vi "VI Reference Based Quadrature.vi"() -> ()   [LabVIEW 2023]
doc: "This example VI shows how to use the Quadrature VI to calculate integrals, and compares the integration results and execution time of 1D Quadrature (VI).vi with the integration results and execution time of 1D Quadrature (Formula).vi."
uses:
  <vilib>/Analysis/1siggen.llb/Ramp Pattern by Samples.vi
  <vilib>/Analysis/8numeric.llb/1D Quadrature (VI).vi
  <vilib>/Analysis/8numeric.llb/1D Quadrature (Formula).vi
  <vilib>/Analysis/NI_AALPro.lvlib
  <vilib>/Analysis/NI_AALBase.lvlib
panel:
  out "Integrand plot":cluster{"Ramp Pattern":dbl[], "F(X)":dbl[]}[](graph)
  out "Time of 1D Quadrature (VI)":u32
  out "Time of 1D Quadrature (Formula)":u32
  out "1D Quadrature (Formula)":dbl
  out "1D Quadrature (VI)":dbl
  in  "term 3":u16(ring) items=["x*x", "x"]
  in  "term 2":u16(ring) items=["cos(0.5*x)", "sin(0.5*x)"]
  in  "term 1":u16(ring) items=["sin(x)", "cos(x)"]
  in  "Lower limit":dbl=-2.0
  in  "Upper limit":dbl=2.0
  # "Overview: Demonstrates how to use the Quadrature VI to calculate integrals.\nRequirements: LabVIEW Full Development System\nInstructions:\n1. Run the VI.\n2. Change the parameters and run the VI again. Integration result indicates that 1D Quadrature (VI).vi and 1D Quadrature (Formula).vi return the same result. Execution time (ms) indicates that 1D Quadrature (VI).vi is much faster than 1D Quadrature (Formula).vi."
  # "Integrand"
  # "+"
  # "-"
  # "Integration result"
  # "Execution time (ms)"
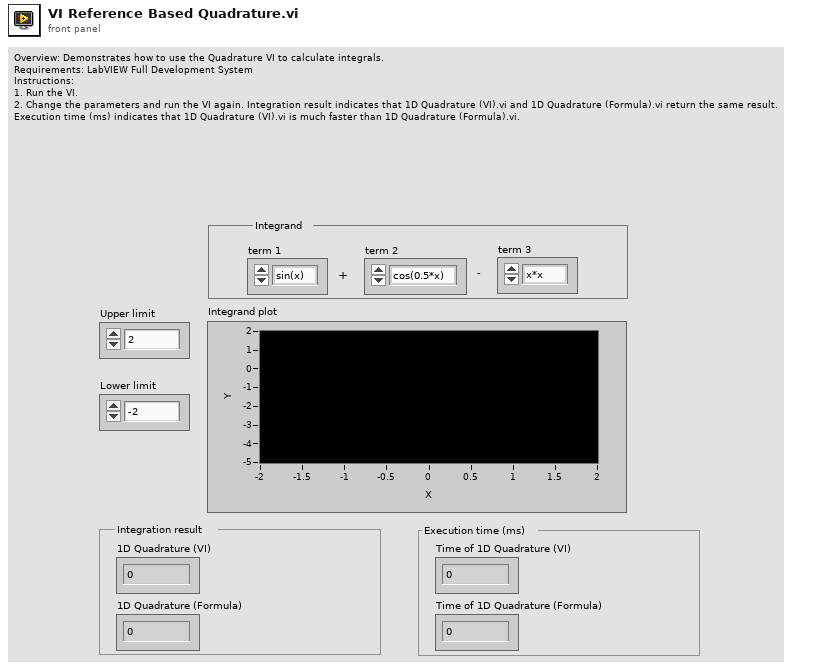
[diagram p1: front panel]
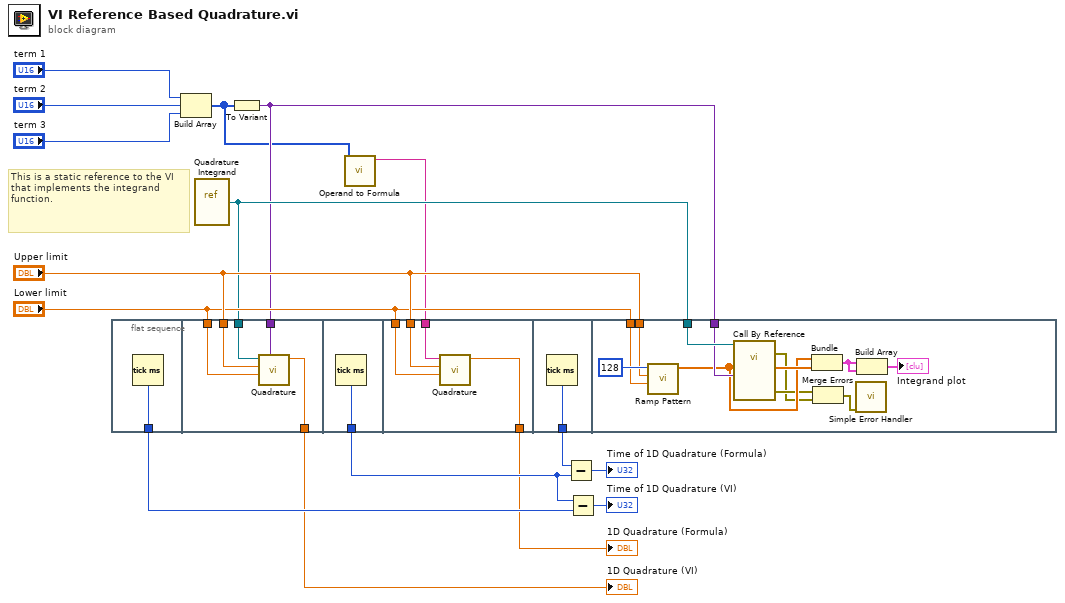
[diagram p0: block diagram]
diagram:
  # "This is a static reference to the VI that implements the integrand function."
  n1 = flat-sequence {
    tunnel: [w17] -> w14
    tunnel: w9 -> [w22]
    tunnel: "Upper limit" -> [w21]
    tunnel: "Lower limit" -> [w20]
    tunnel: [w19] -> w8
    tunnel: w3 -> [w18]
    tunnel: [w23] -> w15
    tunnel: "Upper limit" -> [w27]
    tunnel: "Lower limit" -> [w26]
    tunnel: [w25] -> w7
    tunnel: w1 -> [w24]
    tunnel: [w28] -> w16
    tunnel: "Upper limit" -> [w39]
    tunnel: "Lower limit" -> [w38]
    tunnel: w9 -> [w37]
    tunnel: w3 -> [w36]
    frame #0 {
      n2 = Tick Count (ms)() -> (millisecond timer value=w17:u32)
    }
    frame #1 {
      n3 = call-poly <vilib>:"Quadrature.vi"("data"=w18, "lower limit"=w20, "upper limit"=w21, "integrand"=w22) -> ("result"=w19:dbl)  [unwired: 6 in, 1 out]
    }
    frame #2 {
      n4 = Tick Count (ms)() -> (millisecond timer value=w23:u32)
    }
    frame #3 {
      n5 = call-poly <vilib>:"Quadrature.vi"("lower limit"=w26, "upper limit"=w27, "integrand"=w24) -> ("result"=w25:dbl)  [unwired: 7 in, 1 out]
    }
    frame #4 {
      n6 = Tick Count (ms)() -> (millisecond timer value=w28:u32)
    }
    frame #5 {
      n7 = call-poly <vilib>:"Ramp Pattern.vi"("start"=w38, "end"=w39, "samples"=128) -> ("Ramp Pattern"=w34:dbl[])  [unwired: 7 in, 1 out]
      n8 = call-by-ref "?"(reference=w37, "data"=w36, "X"=w34) -> (error out=w29:errorcluster, 0:"error out"=w30:errorcluster, "F(X)"=w35:dbl[])  [unwired: 9 in, 1 out]
      n9 = Bundle("Ramp Pattern"=w34, "F(X)"=w35) -> (w33:cluster{"Ramp Pattern":dbl[], "F(X)":dbl[]})  [unwired: 1 in]
      n10 = Merge Errors(w30, w29) -> (w31:errorcluster)
      n11 = call <vilib>:"Simple Error Handler.vi"("error in (no error)"=w31) -> ()  [unwired: 4 in, 5 out]
      n12 = Build Array(w33, w33) -> (→"Integrand plot":cluster{"Ramp Pattern":dbl[], "F(X)":dbl[]}[])
    }
  }
  n13 = Build Array("term 1", "term 2", "term 3") -> (w2:u16[])
  n14 = vi-ref "Quadrature Integrand.vi"() -> (w9:refnum<vi>)
  n15 = To Variant(anything=w2) -> (Variant=w3:variant)
  n16 = call "Operand to Formula.vi"("Operand"=w2) -> ("integrand formula"=w1:string)  [unwired: 10 in]
  n17 = Subtract(x=w16, y=w15) -> (x-y=→"Time of 1D Quadrature (Formula)":u32)
  n18 = Subtract(x=w15, y=w14) -> (x-y=→"Time of 1D Quadrature (VI)":u32)
  "1D Quadrature (VI)" <- w8
  "1D Quadrature (Formula)" <- w7
